vi "VI Tree.vi"   [LabVIEW 2014, in "Fluke 190 Series II.lvlib"]
doc: "This is the instrument driver for the Fluke 190 Series II scopemeter (190-062, 190-102,190-104, 190-202, 190-204, 190-502, 190-504). The VI Tree displays all the user-callable VIs of the instrument driver in an organized table."
uses:
  Fluke 190 Series II.lvlib
  Data/Read Measurement (Meter Mode).vi
panel:
  # "(c) 2013-2014 National Instruments.  ALL RIGHTS RESERVED."
  # "SEE DIAGRAM\nFOR VI TREE."
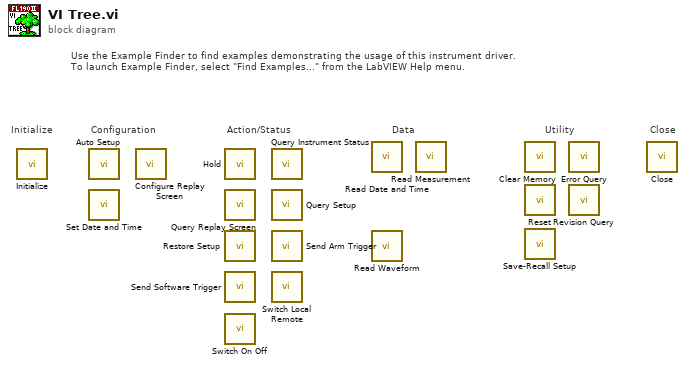
[diagram p0: block diagram]
diagram:
  # "Action/Status"
  # "Use the Example Finder to find examples demonstrating the usage of this instrument driver.\nTo launch Example Finder, select \"Find Examples...\" from the LabVIEW Help menu."
  # "Configuration"
  # "Utility"
  # "Data"
  # "Close"
  # "Initialize"
  n1 = call "Initialize.vi"() -> ()  [unwired: 10 in, 2 out]
  n2 = call "Auto Setup.vi"() -> ()  [unwired: 10 in, 2 out]
  n3 = call "Set Date and Time.vi"() -> ()  [unwired: 10 in, 2 out]
  n4 = call "Configure Replay Screen.vi"() -> ()  [unwired: 10 in, 2 out]
  n5 = call "Hold.vi"() -> ()  [unwired: 10 in, 2 out]
  n6 = call "Query Replay Screen.vi"() -> ()  [unwired: 8 in, 4 out]
  n7 = call "Restore Setup.vi"() -> ()  [unwired: 10 in, 2 out]
  n8 = call "Send Software Trigger.vi"() -> ()  [unwired: 10 in, 2 out]
  n9 = call "Switch On Off.vi"() -> ()  [unwired: 10 in, 2 out]
  n10 = call "Query Instrument Status.vi"() -> ()  [unwired: 9 in, 3 out]
  n11 = call "Query Setup.vi"() -> ()  [unwired: 10 in, 2 out]
  n12 = call "Send Arm Trigger.vi"() -> ()  [unwired: 10 in, 2 out]
  n13 = call "Switch Local Remote.vi"() -> ()  [unwired: 10 in, 2 out]
  n14 = call "Read Date and Time.vi"() -> ()  [unwired: 8 in, 4 out]
  n15 = call "Read Waveform.vi"() -> ()  [unwired: 9 in, 7 out]
  n16 = call-poly "Read Measurement.vi"() -> ()  [unwired: 9 in, 3 out]
  n17 = call "Clear Memory.vi"() -> ()  [unwired: 10 in, 2 out]
  n18 = call "Reset.vi"() -> ()  [unwired: 10 in, 2 out]
  n19 = call "Save-Recall Setup.vi"() -> ()  [unwired: 10 in, 2 out]
  n20 = call "Error Query.vi"() -> ()  [unwired: 8 in, 4 out]
  n21 = call "Revision Query.vi"() -> ()  [unwired: 8 in, 4 out]
  n22 = call "Close.vi"() -> ()  [unwired: 11 in, 1 out]
